vi "PH_DataViewer.set Calorimeter GUI elements.vi"(7 "Calorimeters":T1[](array[typedef]) {"PH Calorimeter Device Config"."Channel Gain" items=["Range: +/- 10 V", "Range: +/- 2.5 V ", "Range: +/- 1 V", "Range: +/- 0.25 V", "Range: +/- 0.1 V", "Range: +/- 0.025 V"]; "PH Calorimeter Device Config"."Channel" items=["Channel 1", "Channel 2", "Channel 3", "Channel 4", "Channel 5", "Channel 6", "Channel 7", "Channel 8", "Channel 9", "Channel 10", "Channel 11", "Channel 12", "Channel 13", "Channel 14", "Channel 15", "Channel 16"]}, 11 "Version":u8) -> (4 "PH Calorimeter Device Config":T2 {"Channel Gain" items=["Range: +/- 10 V", "Range: +/- 2.5 V ", "Range: +/- 1 V", "Range: +/- 0.25 V", "Range: +/- 0.1 V", "Range: +/- 0.025 V"]; "Channel" items=["Channel 1", "Channel 2", "Channel 3", "Channel 4", "Channel 5", "Channel 6", "Channel 7", "Channel 8", "Channel 9", "Channel 10", "Channel 11", "Channel 12", "Channel 13", "Channel 14", "Channel 15", "Channel 16"]}, 6 "Energy [J]":dbl, 8 "Graph Data":cluster{"Raw Data":dbl[], "Raw Data":dbl[]}, 10 "Taken + Calc: Date":string, 15 "Taken + Calc: Time":string)   [LabVIEW 2014, in "PH_DataViewer.lvlib"]
doc: "This VI prepares the information to be indicated."
uses:
  PH_DataViewer.lvlib
  PH_Calorimeter_USB/PH_Calorimeter_USB.Device Config.ctl
  PH_Calorimeter_USB/PH_Calorimeter_USB.Channel.ctl
  PH_Calorimeter_USB/PH_Calorimeter_USB.Channel Gain.ctl
  PH_Calorimater_USB.Data.ctl
  PH_Calorimeter_USB/PH_Calorimeter_USB.lvlib
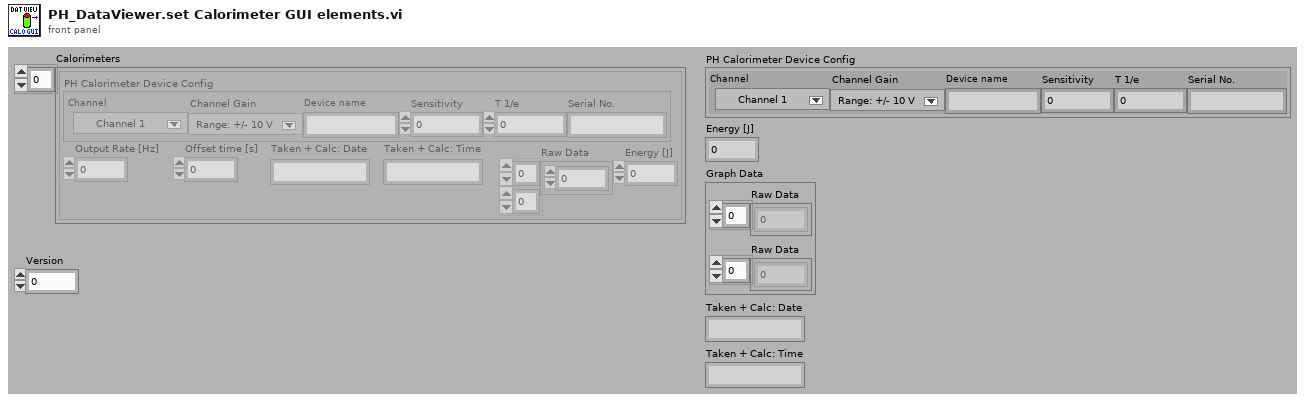
[diagram p1: front panel]
types:
  T1 = typedef "PH_DataViewer.lvlib/PH_Calorimater_USB.Data.ctl" = cluster{"PH Calorimeter Device Config":T2, "Output Rate [Hz]":i32, "Offset time [s]":dbl, "Taken + Calc: Date":string, "Taken + Calc: Time":string, "Raw Data":dbl[][], "Energy [J]":dbl}
  T2 = typedef "PH_Calorimeter_USB.lvlib/PH_Calorimeter_USB.Device Config.ctl" = cluster{"Channel":T3, "Channel Gain":T4, "Device name":string, "Sensitivity":dbl, "T 1/e":dbl, "Serial No.":string}
  T3 = typedef "PH_Calorimeter_USB.lvlib/PH_Calorimeter_USB.Channel.ctl" = u16
  T4 = typedef "PH_Calorimeter_USB.lvlib/PH_Calorimeter_USB.Channel Gain.ctl" = u16
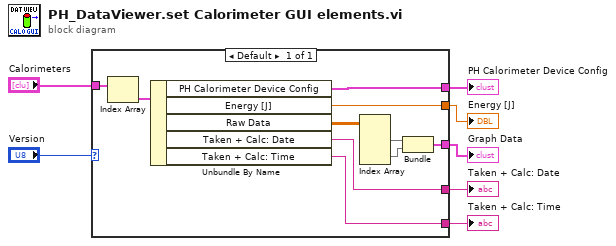
[diagram p0: block diagram]
diagram:
  n1 = case shown="Default" "Version" {
    tunnel: [w17] -> w7
    tunnel: [w16] -> w6
    tunnel: [w15] -> w5
    tunnel: [w12] -> w4
    tunnel: [w11] -> w3
    tunnel: "Calorimeters" -> [w8]
    frame Default {
      n2 = Index Array(array=w8) -> (element=w9:T1)  [unwired: 1 in]
      n3 = Unbundle By Name(w9) -> ("PH Calorimeter Device Config"=w12:T2, "Energy [J]"=w11:dbl, "Raw Data"=w10:dbl[][], "Taken + Calc: Date"=w16:string, "Taken + Calc: Time"=w17:string)
      n4 = Index Array(array=w10) -> (element #1=w13:dbl[], element #2=w14:dbl[])  [unwired: 4 in]
      n5 = Bundle("Raw Data"=w13, "Raw Data"=w14) -> (w15:cluster{"Raw Data":dbl[], "Raw Data":dbl[]})  [unwired: 1 in]
    }
  }
  "Taken + Calc: Time" <- w7
  "Taken + Calc: Date" <- w6
  "Graph Data" <- w5
  "PH Calorimeter Device Config" <- w4
  "Energy [J]" <- w3
